vi "Configure IScan Trigger (Zone).vi"(0 "VISA resource name":refnum<visa-resource-name>, 1 "Enable Zone (F: Disable)":bool, 2 "Mode (0: And Must Intersect)":i32(ring) items=["And Must Intersect", "And Must Not Intersect", "Or Must Interset", "Or Must Not Intersect"], 3 "Zone Number (1: 1)":i32(ring)=1 items=["1"=1, "2"=2, "3"=3, "4"=4], 5 "Channel (1: Channel1)":i32(ring)=1 items=["Channel1"=1, "Channel2"=2, "Channel3"=3, "Channel4"=4], 7 "Height (0 V)":dbl, 9 "Width (0 S)":dbl, 11 "error in (no error)":errorcluster, 12 "X Center (0 S)":dbl, 13 "Y Center (0 V)":dbl) -> (4 "VISA resource name out":refnum<visa-resource-name>, 15 "error out":errorcluster)   [LabVIEW 2020, in "Agilent 90000 Series.lvlib"]
doc: "Configures InfiniiScan trigger under zone trigger mode."
uses:
  Agilent 90000 Series.lvlib
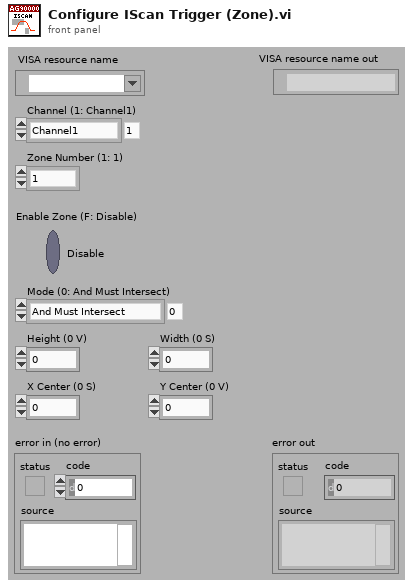
[diagram p1: front panel]
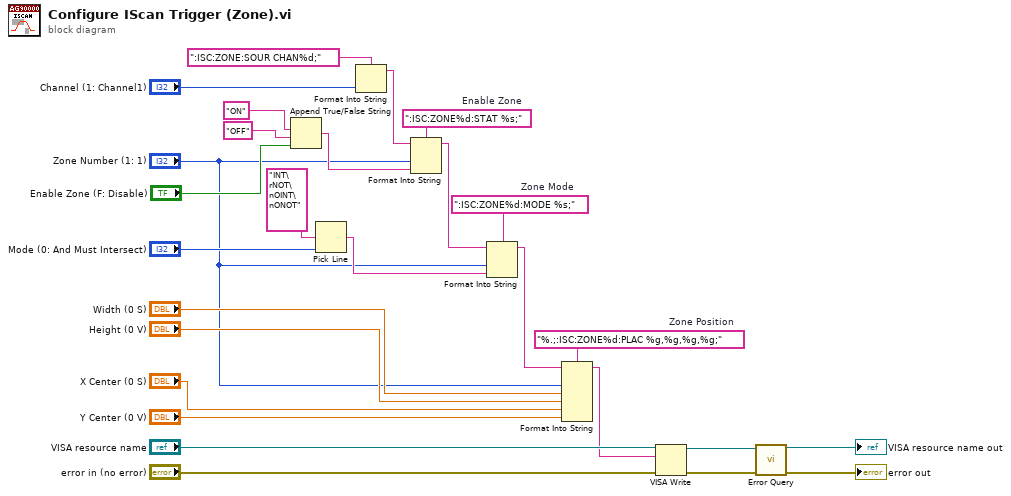
[diagram p0: block diagram]
diagram:
  w13 = ":ISC:ZONE%d:STAT %s;"  # Enable Zone
  w22 = "%.;:ISC:ZONE%d:PLAC %g,%g,%g,%g;"  # Zone Position
  w24 = ":ISC:ZONE%d:MODE %s;"  # Zone Mode
  n1 = Append True/False String(1:"Enable Zone (F: Disable)", 2:"OFF", 3:"ON") -> (0:w12:string)  [unwired: 1 out]
  n2 = Pick Line(multi-line string="INT\rNOT\nOINT\nONOT", line index="Mode (0: And Must Intersect)") -> (output string=w23:string)  [unwired: 1 out]
  n3 = Format Into String(format string=":ISC:ZONE:SOUR CHAN%d;", "Channel (1: Channel1)") -> (resulting string=w3:string)  [unwired: 2 in, 1 out]
  n4 = Format Into String(format string=w13, initial string=w3, "Zone Number (1: 1)", w12) -> (resulting string=w2:string)  [unwired: 1 in, 1 out]
  n5 = Format Into String(format string=w24, initial string=w2, "Zone Number (1: 1)", w23) -> (resulting string=w21:string)  [unwired: 1 in, 1 out]
  n6 = Format Into String(format string=w22, initial string=w21, "Zone Number (1: 1)", "Width (0 S)", "Height (0 V)", "X Center (0 S)", "Y Center (0 V)") -> (resulting string=w1:string)  [unwired: 1 in, 1 out]
  n7 = VISA Write(VISA resource name="VISA resource name", write buffer=w1, error in (no error)="error in (no error)") -> (VISA resource name out=w9:refnum<visa-resource-name>, error out=w8:errorcluster)  [unwired: 1 out]
  n8 = call "Error Query.vi"("error in (no error)"=w8, "VISA resource name"=w9) -> ("error out"=→"error out":errorcluster, "VISA resource name out"=→"VISA resource name out":refnum<visa-resource-name>)  [unwired: 8 out]
